vi "Init.vi"(8 "error in":errorcluster, 11 "Data":variant) -> (0 "error out":errorcluster)   [LabVIEW 2013, in "Error Handler.lvlib"]
doc: "This VI enqueues the named action."
uses:
  Error Handler.lvlib
  Private Controls/Module Data Cluster.ctl
  Private Controls/Module Action.ctl
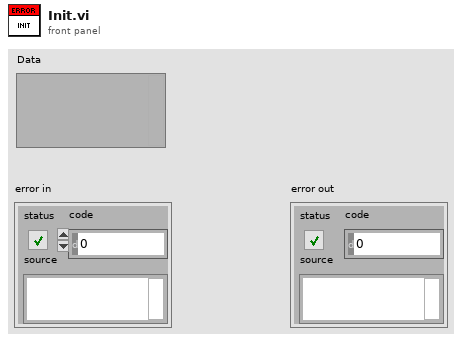
[diagram p1: front panel]
types:
  T1 = typedef "Error Handler.lvlib/Module Data Cluster.ctl" = cluster{"Data":variant, "Action":T2}
  T2 = typedef "Error Handler.lvlib/Module Action.ctl" = enum16{"Process_Step_Err", "Sensor_IO_err", "User_Console_err", "Display_Consol_err", "Error_Log", "Error", "Exit", "Init"}
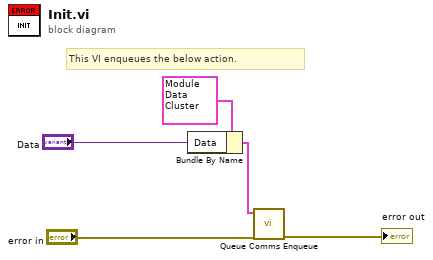
[diagram p0: block diagram]
diagram:
  # "This VI enqueues the below action."
  n1 = Bundle By Name(cluster=T1 {"Data"=variant, "Action"=enum."Init"} ("element"), "Data"="Data") -> (w1:T1)
  n2 = call "Queue Comms Enqueue.vi"("error in"="error in", "element"=w1) -> ("error out"=→"error out":errorcluster)  [unwired: 9 in]
